vi "Vision Research Phantom Series PhInt PhTriplicateGray.vi"(0 "pBMIH":T1, 1 "pPixel [in]":u16[](array[numeric]), 5 "Error In (no error)":errorcluster) -> (14 "pPixel [out]":u16[](array[numeric]), 19 "Error Out":errorcluster)   [LabVIEW 2013, in "VRI.lvlib"]
doc: "PhTriplicateGray\nvoid PhTriplicateGray(PBITMAPINFOHEADER pBMIH, PBYTE pPixel);\n\nParameters\npBMIH \n DIB header.\npPixel\n Pixel array.\n\nNo Return Value\n\nRemarks\nBuild a color RGB image from an monochrome bitmap by copying the same value in the three color component. \nThe input image can be 8 or 16 bit per pixel, the result will be 24 or 48 bpp. \nThe biBitCount and biSizeImage fields of the header are updated. \nThe pPixel array must be allocated for the resulting color image that is three times larger than the original array. \nThis function is needed in Labview.\n\nRequired header\n PhInt.h"
uses:
  VRI.lvlib
  _Type Defs/BITMAPINFOHEADER.ctl
  Phantom DLLs/PhInt.Dll
panel:
  # "For instructions on the use of this VI, press Ctrl+H to display the help window and move the mouse over the icon, controls, and indicators"
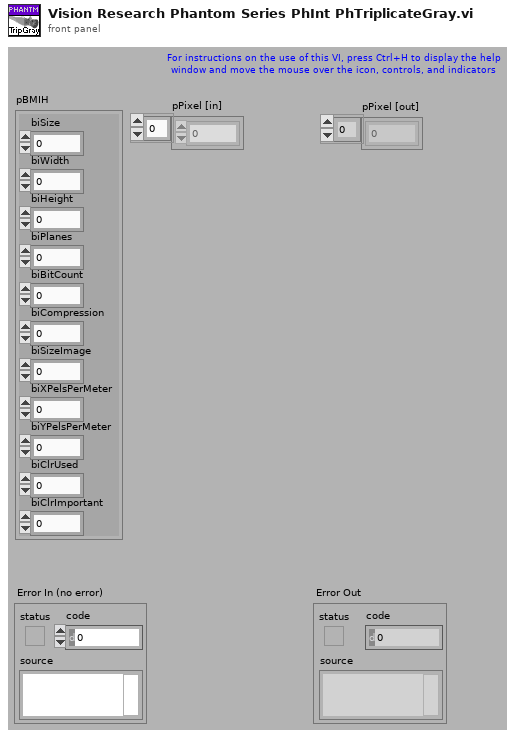
[diagram p1: front panel]
types:
  T1 = typedef "VRI.lvlib/BITMAPINFOHEADER.ctl" = cluster{"biSize":u32, "biWidth":i32, "biHeight":i32, "biPlanes":u16, "biBitCount":u16, "biCompression":u32, "biSizeImage":u32, "biXPelsPerMeter":i32, "biYPelsPerMeter":i32, "biClrUsed":u32, "biClrImportant":u32}
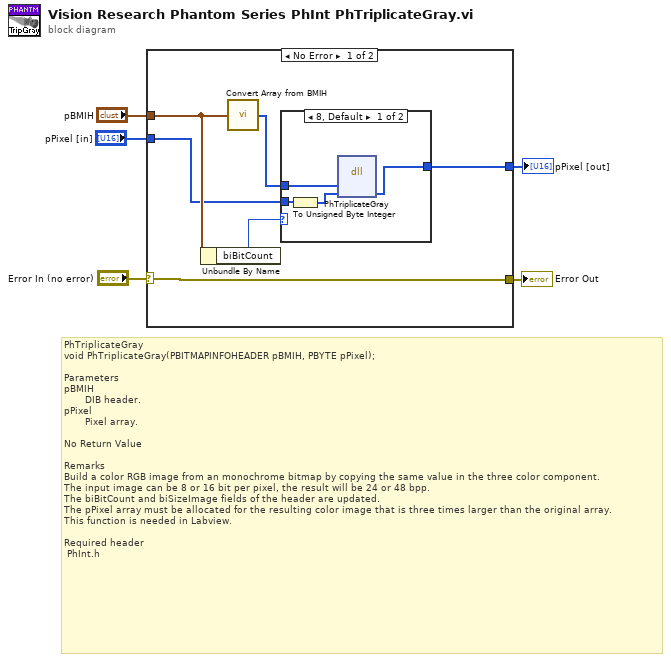
[diagram p0: block diagram]
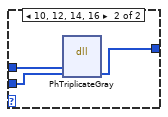
[diagram p2: hidden frame]
diagram:
  # "PhTriplicateGray\nvoid PhTriplicateGray(PBITMAPINFOHEADER pBMIH, PBYTE pPixel);\n\nParameters\npBMIH \n\t      DIB header.\npPixel\n\t      Pixel array.\n\nNo Return Value\n\nRemarks\nBuild a color RGB image from an monochrome bitmap by copying the same value in the three color component. \nThe input image can be 8 or 16 bit per pixel, the result will be 24 or 48 bpp. \nThe biBitCount and biSizeImage fields of the header are updated. \nThe pPixel array must be allocated for the resulting color image that is three times larger than the original array. \nThis function is needed in Labview.\n\nRequired header\n\tPhInt.h"
  n1 = case shown="No Error" "Error In (no error)" {
    selector: "Error In (no error)" -> [w11 w20]
    tunnel: [w11 w20] -> w4
    tunnel: "pBMIH" -> [w10 _]
    tunnel: "pPixel [in]" -> [w9 w19]
    tunnel: [w8 w19] -> w1
    frame No Error {
      n2 = Unbundle By Name(w10) -> ("biBitCount"=w7:u16)
      n3 = call "Convert Array from BMIH.vi"("BITMAPINFOHEADER"=w10) -> ("Array"=w6:u8[])
      n4 = case shown="8, Default" w7 {
        tunnel: w6 -> [w15 w18]
        tunnel: w9 -> [w14 w17]
        tunnel: [w12 w16] -> w8
        frame 8, Default {
          n5 = To Unsigned Byte Integer(number=w14) -> (unsigned 8bit integer=w13:u8[])
          n6 = dll-call lib="C:/Projects/SDK/64-bit/Vision Research Phantom Series Labview Driver/Phantom DLLs/PhInt.dll" fn="PhTriplicateGray"("pBMIH"=w15, "pPixel"=w13) -> ("pPixel"=w12:u8[])  [unwired: 4 in, 3 out]
        }
        frame 10, 12, 14, 16 {
          n7 = dll-call lib="C:/Projects/SDK/64-bit/Vision Research Phantom Series Labview Driver/Phantom DLLs/PhInt.dll" fn="PhTriplicateGray"("pBMIH"=w18, "pPixel"=w17) -> ("pPixel"=w16:u16[])  [unwired: 4 in, 3 out]
        }
      }
    }
    frame Error {
    }
  }
  "Error Out" <- w4
  "pPixel [out]" <- w1
